vi "Datasheet Report Assign Runs to Plots.vi"(0 "Parameters":T8, 5 "Runs for this plot":T5[](array[typedef]), 7 "Preview?":bool, 9 "Template Record":T1, 11 "error in (no error)":errorcluster) -> (1 "sequence":string, 3 "test status":string, 4 "Parameters":T8, 6 "time stamp":string, 10 "operator":string, 12 "Custom Fields":T2[][](array[typedef]), 14 "test station":string, 15 "error out":errorcluster)   [LabVIEW 2011]
uses:
  ITK EXT/utils/keyedarr.llb/Keyed Array.ctl
  TDMS/TDMS File.ctl
  TDMS/TDMS Run.ctl
  TDMS/TDMS Channel (Sxx).ctl
  database/Fields/Field Record.ctl
  database/Fields/Field DataTypes.ctl
  database/Fields/Field NextItem.ctl
  database/Templates/Template Record.ctl
  ITK EXT/utils/strutil.llb/Case Matching.ctl
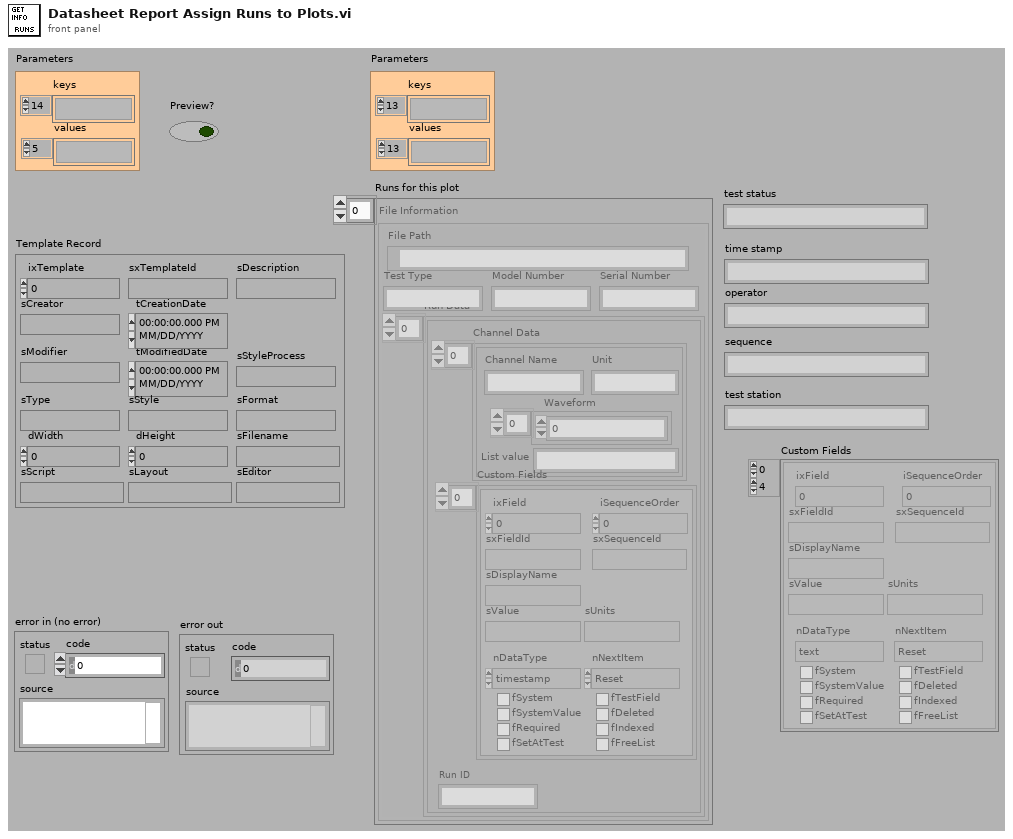
[diagram p1: front panel]
types:
  T1 = typedef "Template Record.ctl" = cluster{"ixTemplate":i32, "sxTemplateId":string, "sDescription":string, "sCreator":string, "tCreationDate":timestamp, "sModifier":string, "tModifiedDate":timestamp, "sType":string, "sStyle":string, "sFormat":string, "dWidth":dbl, "dHeight":dbl, "sFilename":string, "sScript":string, "sLayout":string, "sEditor":string, "sStyleProcess":string}
  T2 = typedef "Field Record.ctl" = cluster{"ixField":i32, "iSequenceOrder":i32, "sxFieldId":string, "sxSequenceId":string, "sDisplayName":string, "sValue":string, "sUnits":string, "nDataType":T3, "nNextItem":T4, "fSystem":bool, "fSystemValue":bool, "fRequired":bool, "fSetAtTest":bool, "fTestField":bool, "fDeleted":bool, "fIndexed":bool, "fFreeList":bool}
  T3 = typedef "Field DataTypes.ctl" = enum32{"text", "numeric", "list", "timestamp", "boolean"}
  T4 = typedef "Field NextItem.ctl" = enum32{"Reset", "Retain", "Auto-Increment"}
  T5 = typedef "TDMS File.ctl" = cluster{"File Path":path, "Run Data":T6[], "Serial Number":string, "Model Number":string, "Test Type":string}
  T6 = typedef "TDMS Run.ctl" = cluster{"Channel Data":T7[], "Custom Fields":T2[], "Run ID":string}
  T7 = typedef "TDMS Channel (Sxx).ctl" = cluster{"Channel Name":string, "Waveform":dbl[], "Unit":string, "List value":string}
  T8 = typedef "Keyed Array.ctl" = cluster{"keys":string[], "values":string[]}
  T9 = typedef "Case Matching.ctl" = enum16{"a != A", "a == A", "system"}
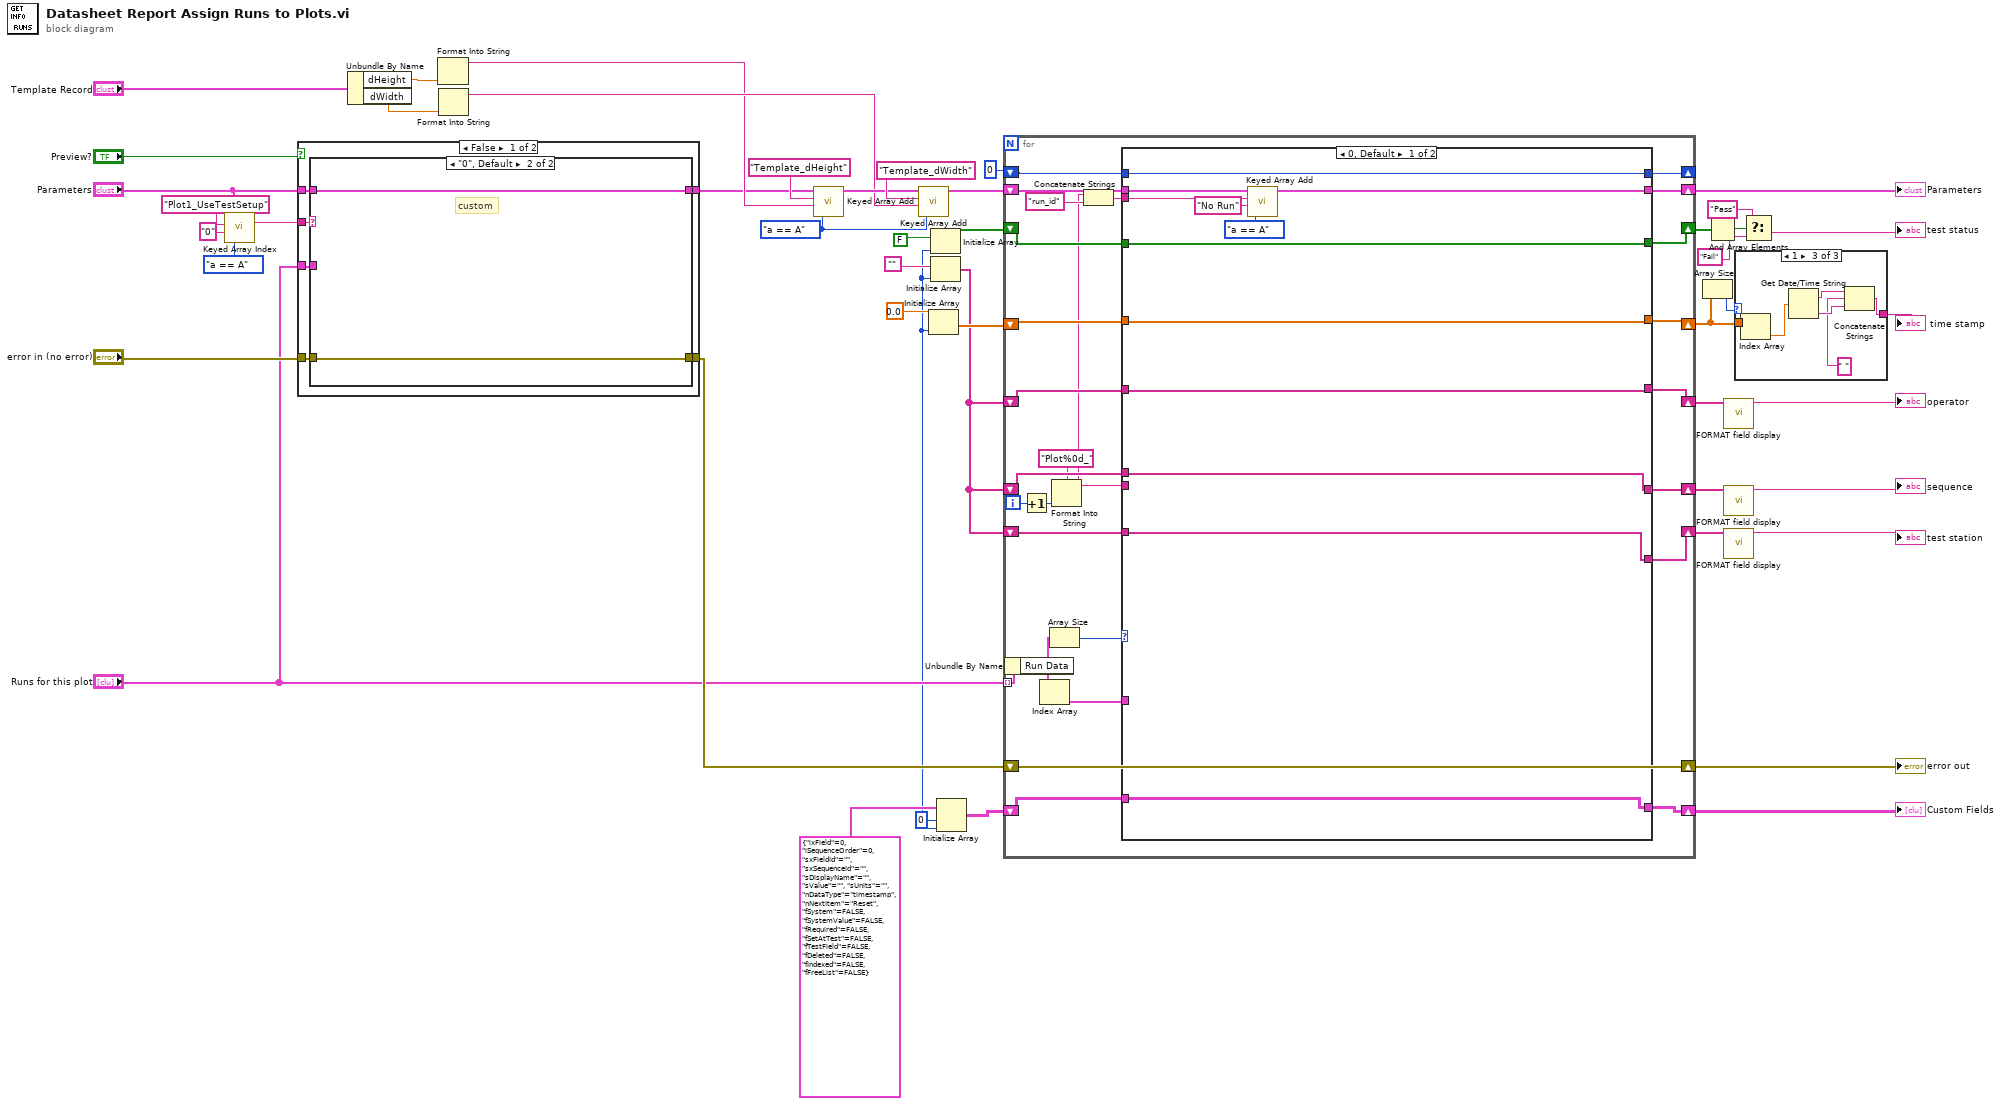
[diagram p0: block diagram]
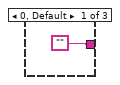
[diagram p2: hidden frame]
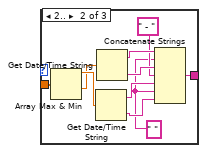
[diagram p3: hidden frame]
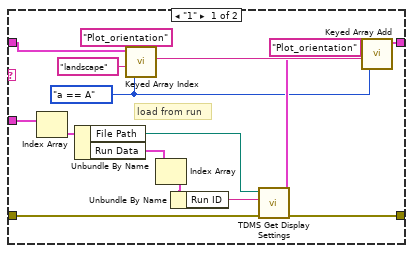
[diagram p4: hidden frame]
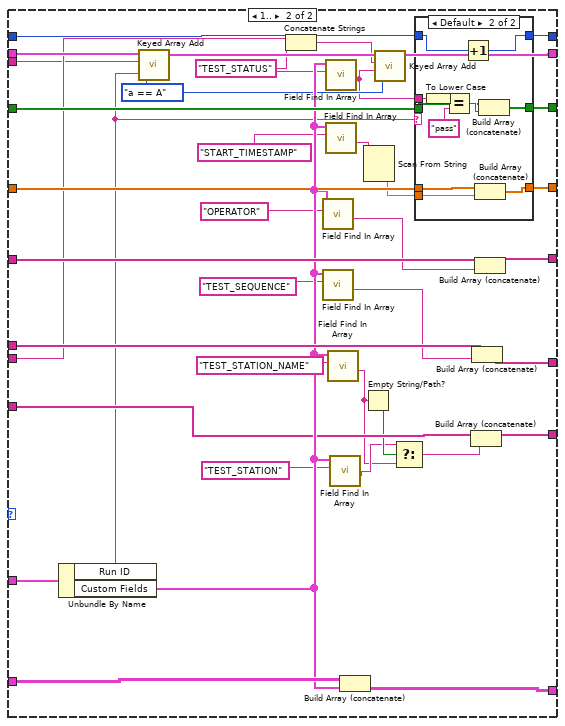
[diagram p6: hidden frame]
diagram:
  w32 = Case_Matching."a == A" ("case matching (sensitive)")
  w8 = 0 ("dimension size")
  n1 = call "Keyed Array Index.vi"("case matching (sensitive)"=Case_Matching."a == A", "default value"="0", "key"="Plot1_UseTestSetup" ("format string"), "array in"="Parameters") -> ("value"=w37:string)  [unwired: 3 out]
  n2 = case shown="False" "Preview?" {
    tunnel: "Runs for this plot" -> [w53 _]
    tunnel: w37 -> [w52 _]
    tunnel: "error in (no error)" -> [w51 w72]
    tunnel: [w50 w73] -> w26
    tunnel: [w49 w72] -> w21
    tunnel: "Parameters" -> [w48 w73]
    frame False {
      n3 = case shown="\"0\", Default" w52 {
        tunnel: w53 -> [w59 _]
        tunnel: w51 -> [w69 w70]
        tunnel: [w68 w70] -> w49
        tunnel: [w66 w71] -> w50
        tunnel: w48 -> [w63 w71]
        frame "1" {
          w60 = Case_Matching."a == A" ("case matching (sensitive)")
          # "load from run"
          n4 = Index Array(array=w59) -> (element=w58:T5)  [unwired: 1 in]
          n5 = Unbundle By Name(w58) -> ("File Path"=w57:path, "Run Data"=w56:T6[])
          n6 = call "Keyed Array Index.vi"("case matching (sensitive)"=w60, "default value"="landscape", "key"="Plot_orientation" ("format string"), "array in"=w63) -> ("value"=w62:string)  [unwired: 3 out]
          n7 = Index Array(array=w56) -> (element=w55:T6)  [unwired: 1 in]
          n8 = Unbundle By Name(w55) -> ("Run ID"=w54:string)
          n9 = call "TDMS Get Display Settings.vi"("error in (no error)"=w69, "Run String"=w54, "TDM File Path"=w57) -> ("error out"=w68:errorcluster, "Parameters"=w61:T8)  [unwired: 7 out]
          n10 = call "Keyed Array Add.vi"("case matching (sensitive)"=w60, "value"=w62, "key"="Plot_orientation" ("format string"), "array in"=w61) -> ("array out"=w66:T8)  [unwired: 3 out]
        }
        frame "0", Default {
          # "custom"
        }
      }
    }
    frame True {
      # "preview"
    }
  }
  n11 = Unbundle By Name("Template Record") -> ("dHeight"=w30:dbl, "dWidth"=w29:dbl)
  n12 = Format Into String(w30) -> (resulting string=w27:string)  [unwired: 3 in, 1 out]
  n13 = Format Into String(w29) -> (resulting string=w28:string)  [unwired: 3 in, 1 out]
  n14 = call "Keyed Array Add.vi"("case matching (sensitive)"=w32, "value"=w27, "key"="Template_dHeight" ("format string"), "array in"=w26) -> ("array out"=w34:T8)  [unwired: 3 out]
  n15 = call "Keyed Array Add.vi"("case matching (sensitive)"=w32, "value"=w28, "key"="Template_dWidth" ("format string"), "array in"=w34) -> ("array out"=w24:T8)  [unwired: 3 out]
  n16 = Initialize Array(0.0, w8) -> (w18:dbl[])
  n17 = Initialize Array(FALSE, w8) -> (w6:bool[])
  n18 = Initialize Array("", w8) -> (w15:string[])
  n19 = Initialize Array(T2 {"ixField"=0, "iSequenceOrder"=0, "sxFieldId"="", "sxSequenceId"="", "sDisplayName"="", "sValue"="", "sUnits"="", "nDataType"=enum."timestamp", "nNextItem"=enum."Reset", "fSystem"=FALSE, "fSystemValue"=FALSE, "fRequired"=FALSE, "fSetAtTest"=FALSE, "fTestField"=FALSE, "fDeleted"=FALSE, "fIndexed"=FALSE, "fFreeList"=FALSE} ("Field Record"), w8, w8) -> (w41:T2[][])
  n20 = for {
    shift-right: [w99] -> w47
    shift-left: w24 -> [w100]
    shift-right: [w98] -> w10
    shift-left: w18 -> [w97]
    shift-right: [w94] -> w44
    shift-left: w15 -> [w93]
    shift-right: [w95] -> w45
    shift-left: w15 -> [w92]
    shift-right: [w96] -> w46
    shift-left: w15 -> [w84]
    shift-right: [w90] -> w5
    shift-left: w6 -> [w91]
    shift-right: [w87] -> w43
    shift-left: w21 -> [w87]
    shift-right: [w89] -> w42
    shift-left: w41 -> [w88]
    tunnel: "Runs for this plot" -> [w85] mode=indexing
    shift-right: [w80] -> _
    shift-left: 0 -> [w81]
    i -> [w76]
    n21 = Unbundle By Name(w85) -> ("Run Data"=w83:T6[])
    n22 = Increment(x=w76) -> (x+1=w79:i32)
    n23 = Index Array(array=w83) -> (element=w86:T6)  [unwired: 1 in]
    n24 = Array Size(array=w83) -> (size(s)=w82:i32)
    n25 = Format Into String(format string="Plot%0d_", w79) -> (resulting string=w74:string)  [unwired: 2 in, 1 out]
    n26 = Concatenate Strings(w74, "run_id" ("format string")) -> (w75:string)
    n27 = case shown="0, Default" w82 {
      tunnel: w100 -> [w105 w151]
      tunnel: [w104 w119] -> w99
      tunnel: [w111 w150] -> w98
      tunnel: w97 -> [w111 w149]
      tunnel: [w108 w148] -> w96
      tunnel: [w109 w147] -> w95
      tunnel: [w110 w146] -> w94
      tunnel: w93 -> [w110 w145]
      tunnel: w92 -> [w109 w144]
      tunnel: w91 -> [w112 w143]
      tunnel: [w112 w142] -> w90
      tunnel: [w107 w141] -> w89
      tunnel: w88 -> [w107 w140]
      tunnel: w86 -> [_ w139]
      tunnel: w84 -> [w108 w137]
      tunnel: w81 -> [w106 w136]
      tunnel: [w106 w121] -> w80
      tunnel: w74 -> [_ w114]
      tunnel: w75 -> [w102 w113]
      frame 0, Default {
        n28 = call "Keyed Array Add.vi"("case matching (sensitive)"=Case_Matching."a == A", "value"="No Run", "key"=w102, "array in"=w105) -> ("array out"=w104:T8)  [unwired: 3 out]
      }
      frame 1.. {
        w118 = Case_Matching."a == A" ("case matching (sensitive)")
        w116 = "TEST_STATUS"
        n29 = Unbundle By Name(w139) -> ("Run ID"=w122:string, "Custom Fields"=w138:T2[])
        n30 = call "Keyed Array Add.vi"("case matching (sensitive)"=w118, "value"=w122, "key"=w113, "array in"=w151) -> ("array out"=w120:T8)  [unwired: 3 out]
        n31 = Concatenate Strings(w114, w116) -> (w115:string)
        n32 = call "Field Find In Array.vi"("FieldID or Display Name(\"\")"="OPERATOR", "Field Array"=w138) -> ("sValue"=w125:string)  [unwired: 1 in, 8 out]
        n33 = call "Field Find In Array.vi"("FieldID or Display Name(\"\")"="TEST_SEQUENCE", "Field Array"=w138) -> ("sValue"=w124:string)  [unwired: 1 in, 8 out]
        n34 = call "Field Find In Array.vi"("FieldID or Display Name(\"\")"=w116, "Field Array"=w138) -> ("sValue"=w117:string)  [unwired: 1 in, 8 out]
        n35 = call "Field Find In Array.vi"("FieldID or Display Name(\"\")"="START_TIMESTAMP", "Field Array"=w138) -> ("sValue"=w127:string)  [unwired: 1 in, 8 out]
        n36 = call "Field Find In Array.vi"("FieldID or Display Name(\"\")"="TEST_STATION_NAME", "Field Array"=w138) -> ("sValue"=w128:string)  [unwired: 1 in, 8 out]
        n37 = call "Field Find In Array.vi"("FieldID or Display Name(\"\")"="TEST_STATION", "Field Array"=w138) -> ("sValue"=w129:string)  [unwired: 1 in, 8 out]
        n38 = Build Array (concatenate)(w140, w138) -> (w141:T2[][])
        n39 = Empty String/Path?(string/path=w128) -> (empty?=w130:bool)
        n40 = Scan From String(input string=w127) -> (output 1=w126:dbl)  [unwired: 3 in, 4 out]
        n41 = call "Keyed Array Add.vi"("case matching (sensitive)"=w118, "value"=w117, "key"=w115, "array in"=w120) -> ("array out"=w119:T8)  [unwired: 3 out]
        n42 = Select(t=w129, s=w130, f=w128) -> (s? t:f=w123:string)
        n43 = case shown="Default" w122 {
          tunnel: [w154 w165] -> w150
          tunnel: w149 -> [w154 w164]
          tunnel: w143 -> [w153 w156]
          tunnel: [w153 w155] -> w142
          tunnel: w136 -> [w152 w161]
          tunnel: w117 -> [_ w163]
          tunnel: w126 -> [_ w162]
          tunnel: [w152 w160] -> w121
          frame "" {
          }
          frame Default {
            n44 = To Lower Case(string=w163) -> (all lower case string=w158:string)
            n45 = Equal?(x=w158, y="pass") -> (x = y?=w157:bool)
            n46 = Increment(x=w161) -> (x+1=w160:i32)
            n47 = Build Array (concatenate)(w164, w162) -> (w165:dbl[])
            n48 = Build Array (concatenate)(w156, w157) -> (w155:bool[])
          }
        }
        n49 = Build Array (concatenate)(w137, w123) -> (w148:string[])
        n50 = Build Array (concatenate)(w144, w124) -> (w147:string[])
        n51 = Build Array (concatenate)(w145, w125) -> (w146:string[])
      }
    }
  }
  "Parameters" <- w47
  "Custom Fields" <- w42
  "error out" <- w43
  n52 = Array Size(array=w10) -> (size(s)=w9:i32)
  n53 = And Array Elements(Boolean array=w5) -> (logical AND=w4:bool)
  n54 = call "FORMAT field display.vi"("strings"=w44) -> ("String"=→"operator":string)  [unwired: 10 out]
  n55 = call "FORMAT field display.vi"("strings"=w45) -> ("String"=→"sequence":string)  [unwired: 10 out]
  n56 = call "FORMAT field display.vi"("strings"=w46) -> ("String"=→"test station":string)  [unwired: 10 out]
  n57 = case shown="1" w9 {
    tunnel: w10 -> [_ w176 w178]
    tunnel: ["" w167 w179] -> w17
    frame 0, Default {
    }
    frame 2.. {
      w168 = " " ("format string")
      n58 = Array Max & Min(array=w176) -> (max value=w175:dbl, min value=w174:dbl)  [unwired: 2 out]
      n59 = Get Date/Time String(seconds (now)=w175) -> (date string=w170:string, time string=w169:string)  [unwired: 2 out]
      n60 = Get Date/Time String(seconds (now)=w174) -> (date string=w173:string, time string=w172:string)  [unwired: 2 out]
      n61 = Concatenate Strings(w173, w168, w172, " - " ("format string"), w170, w168, w169) -> (w167:string)
    }
    frame 1 {
      n62 = Index Array(array=w178) -> (element=w177:dbl)  [unwired: 1 in]
      n63 = Get Date/Time String(seconds (now)=w177) -> (date string=w182:string, time string=w181:string)  [unwired: 2 out]
      n64 = Concatenate Strings(w182, " " ("format string"), w181) -> (w179:string)
    }
  }
  "time stamp" <- w17
  n65 = Select(t="Pass", s=w4, f="Fail") -> (s? t:f=→"test status":string)
